vi "Set Player Ship.vi"(8 "error in (no error)":errorcluster, 10 "Ship":T1, 11 "Player":T2) -> (0 "error out":errorcluster)   [LabVIEW 2015, in "Main Controller Actor API.lvclass"]
uses:
  Main Controller Actor API.lvclass
  Controls/Player.ctl
  Controls/Ship.ctl
  Actor/Player Ship.ctl
  Re-use Libraries/Minimal Actor Framework/Messaging/Message/Message.lvclass/Message.ctl
  Globals.vi
  Re-use Libraries/Minimal Actor Framework/Messaging/Message/Message.lvclass
  Actor/Main Controller Actor.lvclass
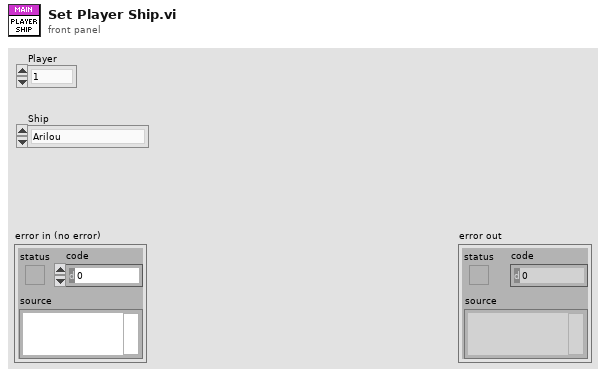
[diagram p1: front panel]
types:
  T1 = typedef "Ship.ctl" = enum16{"Arilou", "Chmmr", "Kohrah"}
  T2 = typedef "Player.ctl" = enum16{"1", "2"}
  T3 = typedef "Main Controller Actor.lvclass/Player Ship.ctl" = cluster{"Player":T2, "Ship":T1}
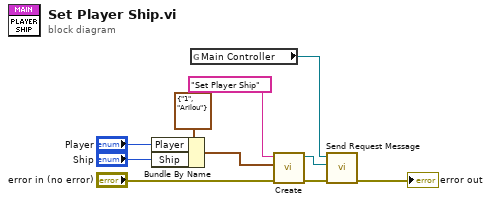
[diagram p0: block diagram]
diagram:
  n1 = Bundle By Name(cluster=T3 {"Player"=enum."1", "Ship"=enum."Arilou"} ("Cluster"), "Player"="Player", "Ship"="Ship") -> (w3:T3)
  n2 = global read "Globals.vi" "Main Controller"() -> (w7:refnum<class "Main Controller Actor API.lvclass">)
  n3 = call "Create.vi"("error in (no error)"="error in (no error)", "Data"=w3, "Name"="Set Player Ship" ("Parameter")) -> ("error out"=w8:errorcluster, "Message out"=w9:refnum<class "Message.lvclass">)  [unwired: 7 in]
  n4 = call-dynamic "Send Request Message.vi"("error in (no error)"=w8, "Message"=w9, "Actor API in"=w7) -> ("error out"=→"error out":errorcluster)  [unwired: 8 in]
